vi "uTTA_FlushSerialBuffer.vi"(4 "error in (no error)":errorcluster, 7 "VISA Refnum in":refnum<visa-resource-name>) -> (0 "error out":errorcluster, 3 "VISA Refnum out":refnum<visa-resource-name>)   [LabVIEW 2021]
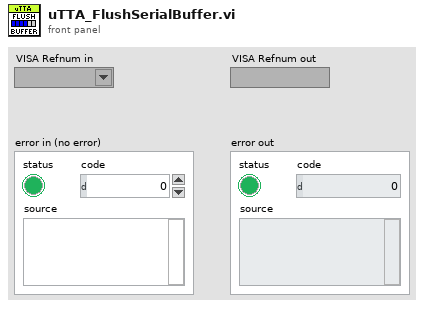
[diagram p1: front panel]
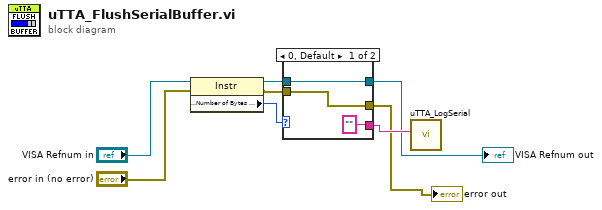
[diagram p0: block diagram]
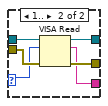
[diagram p2: hidden frame]
diagram:
  n1 = property class="Instr"(reference="VISA Refnum in", error in="error in (no error)") -> (reference out=w1:refnum<visa-resource-name>, error out=w2:errorcluster, "Serial Settings:Number of Bytes at Serial Port"=w3:u32)
  n2 = case shown="0, Default" w3 {
    selector: w3 -> [_ w15]
    tunnel: w1 -> [w11 w17]
    tunnel: w2 -> [w10 w16]
    tunnel: [w11 w14] -> w6
    tunnel: [w10 w13] -> w7
    tunnel: ["" ("read buffer") w12] -> w8
    frame 0, Default {
    }
    frame 1.. {
      n3 = VISA Read(VISA resource name=w17, byte count=w15, error in (no error)=w16) -> (VISA resource name out=w14:refnum<visa-resource-name>, read buffer=w12:string, error out=w13:errorcluster)  [unwired: 1 out]
    }
  }
  "error out" <- w7
  "VISA Refnum out" <- w6
  n4 = call "uTTA_LogSerial.vi"("Data_Sent"=w8) -> ()  [unwired: 6 in, 1 out]
